vi "Check Redlines.vi"(8 "error in (no error)":errorcluster, 9 "Data":dbl[][](array[numeric]), 11 "DataProcessor in":refnum<class "DataProcessor.lvclass">) -> (0 "error out":errorcluster, 3 "DataProcessor out":refnum<class "DataProcessor.lvclass">)   [LabVIEW 2020, in "Volatus.lvlib" / "DataProcessor.lvclass"]
uses:
  DataProcessor.lvclass
  DataProcessor.lvclass/DataProcessor.ctl
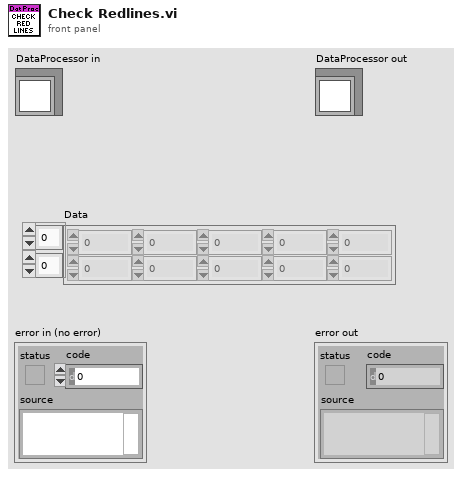
[diagram p1: front panel]
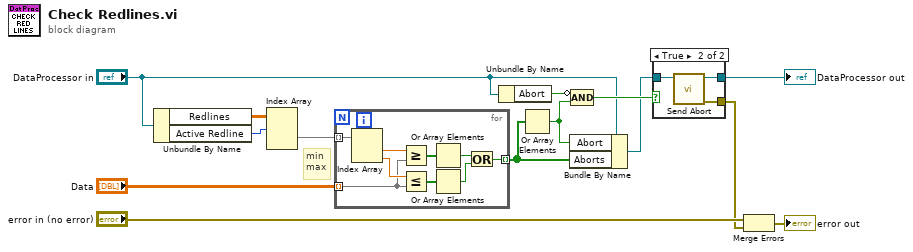
[diagram p0: block diagram]
diagram:
  # "min\nmax"
  n1 = Unbundle By Name("DataProcessor in") -> ("Redlines"=w3:dbl[][][], "Active Redline"=w2:i32)
  n2 = Index Array(array=w3, index (dim 0)=w2) -> (element=w1:dbl[][])  [unwired: 2 in]
  n3 = for {
    tunnel: w1 -> [w23] mode=indexing
    tunnel: "Data" -> [w20] mode=indexing
    tunnel: [w15] -> w12 mode=indexing
    n4 = Index Array(array=w23) -> (element #1=w22:dbl, element #2=w21:dbl)  [unwired: 2 in]
    n5 = Greater Or Equal?(x=w22, y=w20) -> (x >= y?=w19:bool[])
    n6 = Less Or Equal?(x=w21, y=w20) -> (x <= y?=w18:bool[])
    n7 = Or Array Elements(Boolean array=w19) -> (logical OR=w17:bool)
    n8 = Or Array Elements(Boolean array=w18) -> (logical OR=w16:bool)
    n9 = Or(x=w17, y=w16) -> (x .or. y?=w15:bool)
  }
  n10 = Unbundle By Name("DataProcessor in") -> ("Abort"=w11:bool)
  n11 = Or Array Elements(Boolean array=w12) -> (logical OR=w10:bool)
  n12 = Bundle By Name(cluster="DataProcessor in", "Abort"=w10, "Aborts"=w12) -> (w5:refnum<class "DataProcessor.lvclass">)
  n13 = Compound Arithmetic op=AND(invert w11, w10) -> (w9:bool)
  n14 = case shown="True" w9 {
    tunnel: [_ w25] -> w7
    tunnel: [w24 w27] -> w6
    tunnel: w5 -> [w24 w26]
    frame False {
    }
    frame True {
      n15 = call "Send Abort.vi"("DataProcessor in"=w26) -> ("error out"=w25:errorcluster, "DataProcessor out"=w27:refnum<class "DataProcessor.lvclass">)  [unwired: 9 in]
    }
  }
  "DataProcessor out" <- w6
  n16 = Merge Errors("error in (no error)", w7) -> (→"error out":errorcluster)
